vi "error_check_spin_diode.vi"(8 "State":T1=enum."Shutdown", 11 "Boolean":bool) -> (2 "Result state":T1)   [LabVIEW 2017]
uses:
  controls/State.ctl
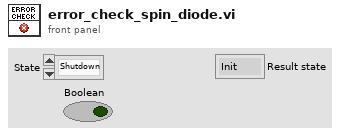
[diagram p1: front panel]
types:
  T1 = typedef "State.ctl" = enum16{"Init", "Idle", "Starting", "Measure", "Stopping", "Shutdown"}
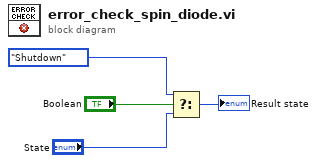
[diagram p0: block diagram]
diagram:
  n1 = Select(t=State."Shutdown", s="Boolean", f="State") -> (s? t:f=→"Result state":T1)
